vi "Actividad 2 - Escritura.vi"() -> ()   [LabVIEW 2020]
uses:
  <vilib>/httpClient/PUTBuffer.vi
  <vilib>/httpClient/LabVIEWHTTPClient.lvlib
panel:
  in  "Fecha":string
  in  "Horizontal Pointer Slide":dbl(slide) scale=0.0..10.0
  in  "Vertical Pointer Slide":dbl(slide) scale=0.0..10.0
  in  "Lateral":bool
  in  "Frontal":bool
  out "error out":errorcluster
  in  "stop 2":bool
  out "body PUT":string
  out "headers PUT":string
  out "error PUT":errorcluster
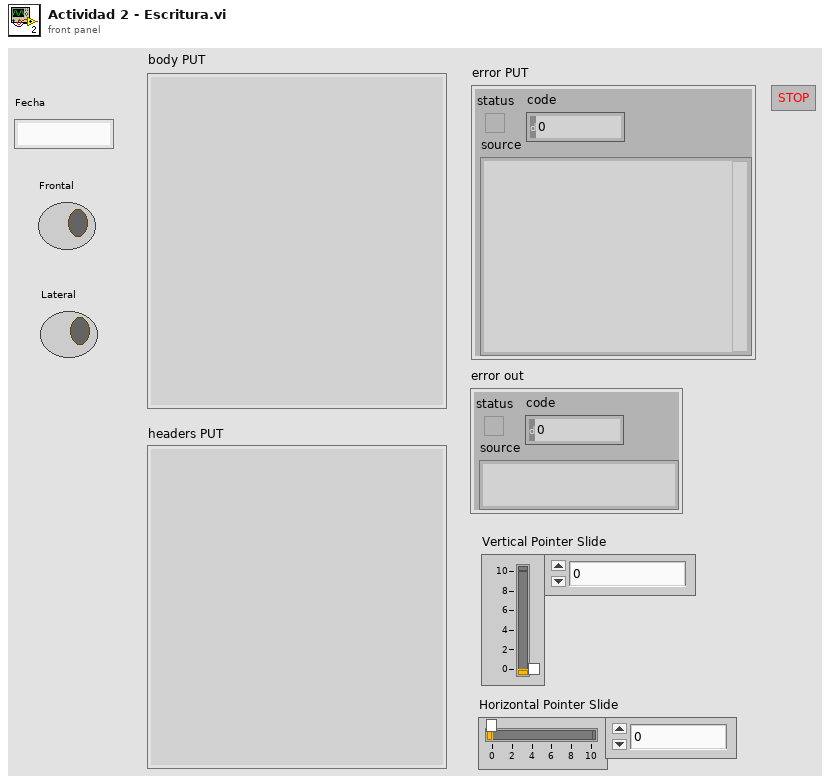
[diagram p1: front panel]
types:
  T1 = cluster{"Humedad":dbl, "Fecha":string, "Temperatura":dbl}
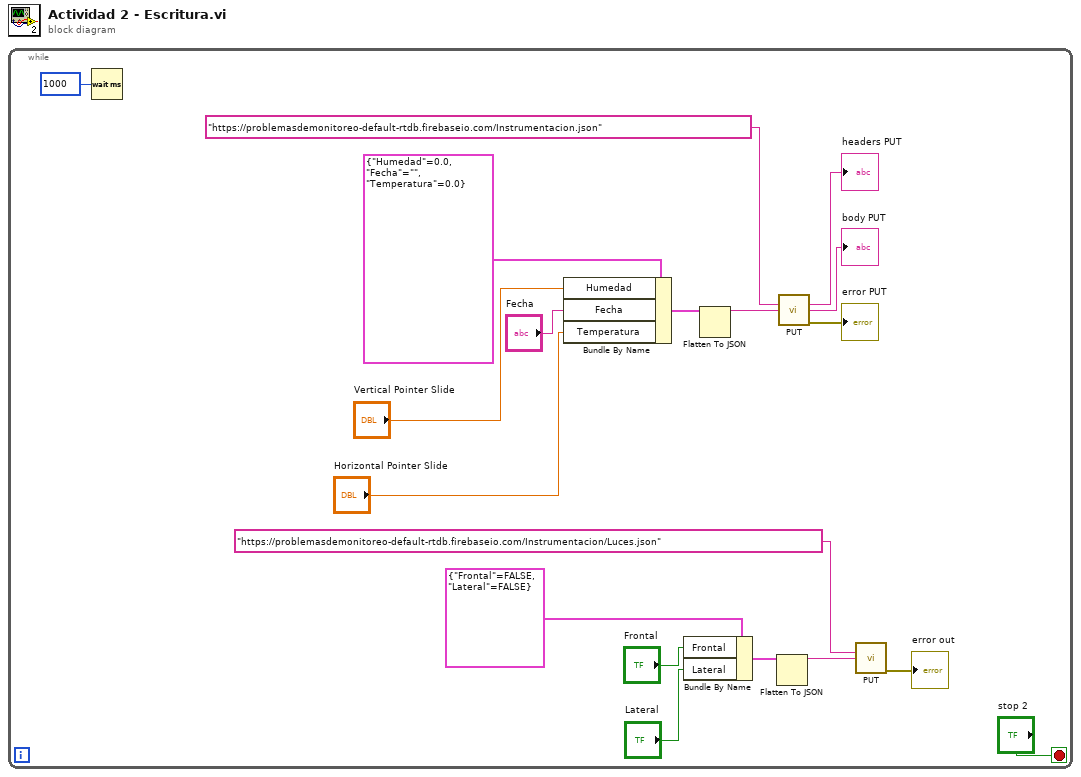
[diagram p0: block diagram]
diagram:
  n1 = while {
    stop <- "stop 2" stop-if-true
    n2 = Wait (ms)(milliseconds to wait=u32 1000) -> ()  [unwired: 1 out]
    n3 = Bundle By Name(cluster=T1 {"Humedad"=0.0, "Fecha"="", "Temperatura"=0.0}, "Humedad"="Vertical Pointer Slide", "Fecha"="Fecha", "Temperatura"="Horizontal Pointer Slide") -> (w12:T1)
    n4 = Bundle By Name(cluster=cluster{"Frontal":bool, "Lateral":bool} {"Frontal"=FALSE, "Lateral"=FALSE}, "Frontal"="Frontal", "Lateral"="Lateral") -> (w3:cluster{"Frontal":bool, "Lateral":bool})
    n5 = Flatten To JSON(anything=w12) -> (JSON string=w18:string)  [unwired: 2 in, 1 out]
    n6 = Flatten To JSON(anything=w3) -> (JSON string=w4:string)  [unwired: 2 in, 1 out]
    n7 = call-poly <vilib>:"PUT.vi"("url"="https://problemasdemonitoreo-default-rtdb.firebaseio.com/Instrumentacion.json", "buffer"=w18) -> ("headers"=→"headers PUT":string, "body"=→"body PUT":string, "error out"=→"error PUT":errorcluster)  [unwired: 10 in, 1 out]
    n8 = call-poly <vilib>:"PUT.vi"("url"="https://problemasdemonitoreo-default-rtdb.firebaseio.com/Instrumentacion/Luces.json", "buffer"=w4) -> ("error out"=→"error out":errorcluster)  [unwired: 10 in, 3 out]
  }
